vi "Test Validation of CLI arguments.vi"() -> (0 "error out":errorcluster)   [LabVIEW 2025]
doc: "Tests validation of CLI arguments."
uses:
  src/Type Definitions/CLI Argument Setting--cluster.ctl
  <vilib>/addons/_JKI Toolkits/Caraya/classes/Test/Test.lvclass
  <vilib>/addons/_JKI Toolkits/Caraya/classes/Assert/Assert.lvclass
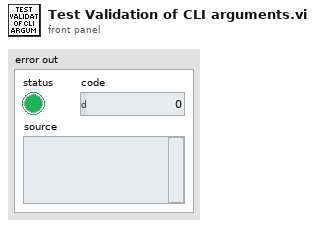
[diagram p1: front panel]
types:
  T1 = typedef "CLI Argument Setting--cluster.ctl" = cluster{"Name Set":bool, "Version Set":bool, "Architecture Set":bool, "File Set":bool}
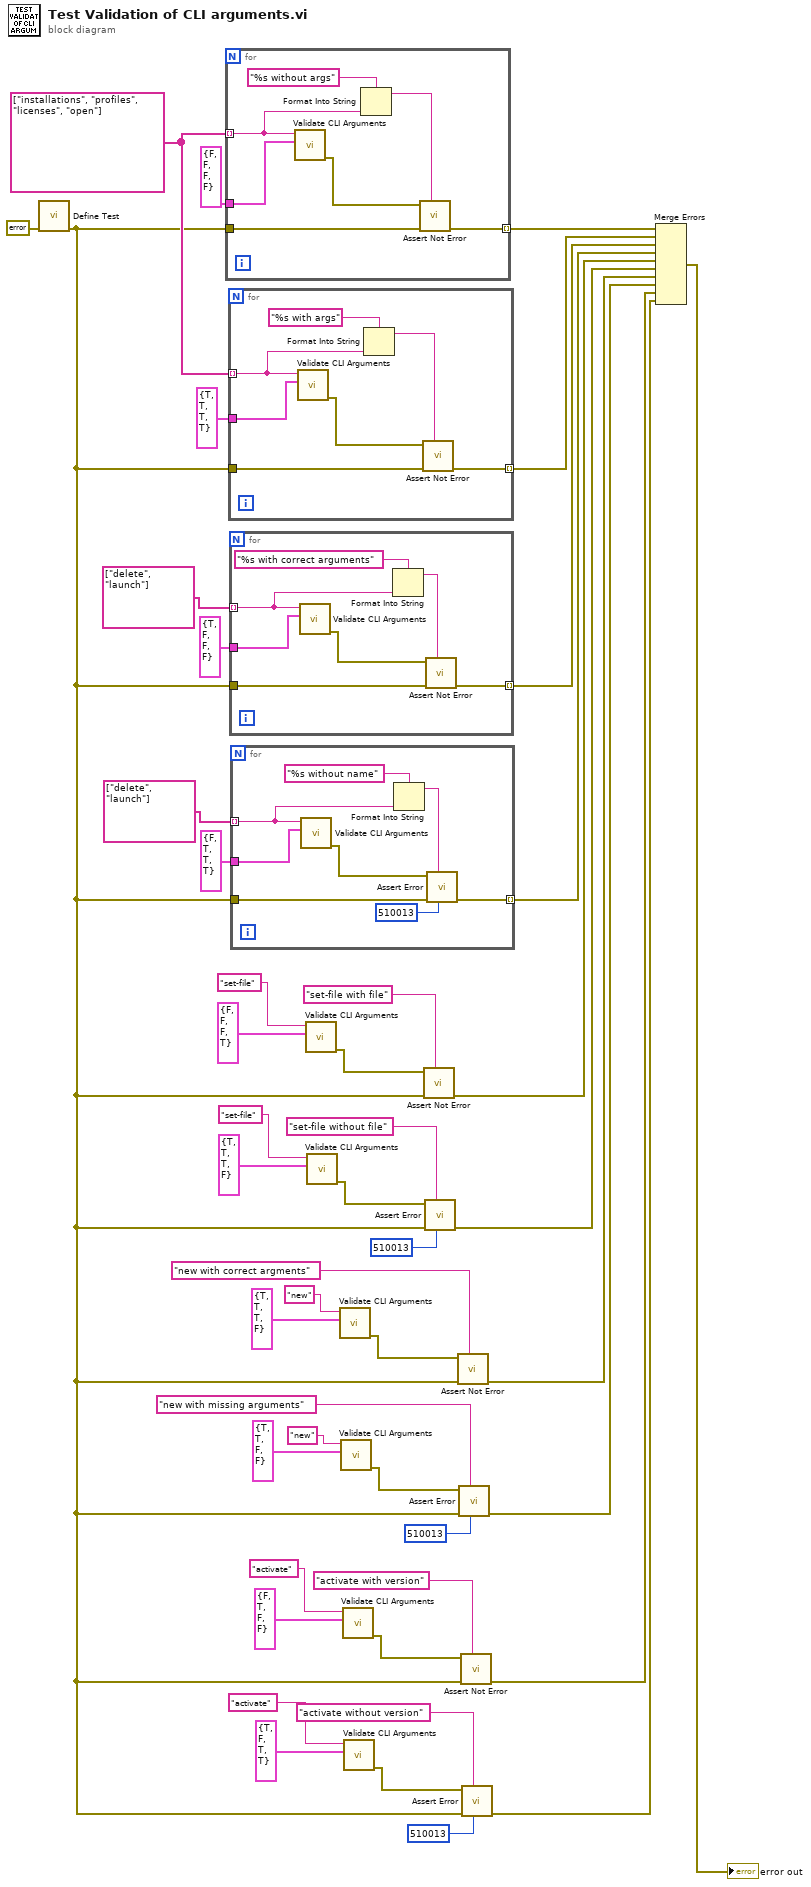
[diagram p0: block diagram]
diagram:
  w46 = string[] ["installations", "profiles", "licenses", "open"]
  n1 = call <vilib>:"Define Test.vi"("error in (no error)"=errorcluster {"status"=FALSE, "code"=0, "source"=""}) -> ("error out"=w3:errorcluster)  [unwired: 9 in, 1 out]
  n2 = for {
    tunnel: w46 -> [w53] mode=indexing
    tunnel: w3 -> [w51]
    tunnel: [w50] -> w26 mode=indexing
    tunnel: T1 {"Name Set"=FALSE, "Version Set"=FALSE, "Architecture Set"=FALSE, "File Set"=FALSE} ("CLI Arguments Setting") -> [w48]
    n3 = call "Validate CLI Arguments.vi"("CLI Arguments Setting"=w48, "Command"=w53) -> ("error out"=w52:errorcluster)  [unwired: 9 in]
    n4 = Format Into String(format string="%s without args" ("Label (VI Title)"), w53) -> (resulting string=w49:string)  [unwired: 2 in, 1 out]
    n5 = call <vilib>:"Assert Not Error.vi"("Label"=w49, "error in (no error)"=w51, "Not Error?"=w52) -> ("error out"=w50:errorcluster)  [unwired: 7 in, 1 out]
  }
  n6 = for {
    tunnel: w46 -> [w60] mode=indexing
    tunnel: w3 -> [w58]
    tunnel: [w57] -> w27 mode=indexing
    tunnel: T1 {"Name Set"=TRUE, "Version Set"=TRUE, "Architecture Set"=TRUE, "File Set"=TRUE} ("CLI Arguments Setting") -> [w55]
    n7 = call "Validate CLI Arguments.vi"("CLI Arguments Setting"=w55, "Command"=w60) -> ("error out"=w59:errorcluster)  [unwired: 9 in]
    n8 = Format Into String(format string="%s with args" ("Label (VI Title)"), w60) -> (resulting string=w56:string)  [unwired: 2 in, 1 out]
    n9 = call <vilib>:"Assert Not Error.vi"("Label"=w56, "error in (no error)"=w58, "Not Error?"=w59) -> ("error out"=w57:errorcluster)  [unwired: 7 in, 1 out]
  }
  n10 = for {
    tunnel: string[] ["delete", "launch"] ("Command") -> [w66] mode=indexing
    tunnel: w3 -> [w64]
    tunnel: [w63] -> w28 mode=indexing
    tunnel: T1 {"Name Set"=TRUE, "Version Set"=FALSE, "Architecture Set"=FALSE, "File Set"=FALSE} ("CLI Arguments Setting") -> [w62]
    n11 = call "Validate CLI Arguments.vi"("CLI Arguments Setting"=w62, "Command"=w66) -> ("error out"=w68:errorcluster)  [unwired: 9 in]
    n12 = Format Into String(format string="%s with correct arguments" ("Label"), w66) -> (resulting string=w65:string)  [unwired: 2 in, 1 out]
    n13 = call <vilib>:"Assert Not Error.vi"("Label"=w65, "error in (no error)"=w64, "Not Error?"=w68) -> ("error out"=w63:errorcluster)  [unwired: 7 in, 1 out]
  }
  n14 = for {
    tunnel: string[] ["delete", "launch"] ("Command") -> [w74] mode=indexing
    tunnel: w3 -> [w72]
    tunnel: [w71] -> w29 mode=indexing
    tunnel: T1 {"Name Set"=FALSE, "Version Set"=TRUE, "Architecture Set"=TRUE, "File Set"=TRUE} ("CLI Arguments Setting") -> [w70]
    n15 = call "Validate CLI Arguments.vi"("CLI Arguments Setting"=w70, "Command"=w74) -> ("error out"=w76:errorcluster)  [unwired: 9 in]
    n16 = Format Into String(format string="%s without name" ("Label"), w74) -> (resulting string=w73:string)  [unwired: 2 in, 1 out]
    n17 = call <vilib>:"Assert Error.vi"("error code (1)"=510013, "Label"=w73, "error in (no error)"=w72, "Error?"=w76) -> ("error out"=w71:errorcluster)  [unwired: 6 in, 1 out]
  }
  n18 = call "Validate CLI Arguments.vi"("CLI Arguments Setting"=T1 {"Name Set"=FALSE, "Version Set"=FALSE, "Architecture Set"=FALSE, "File Set"=TRUE}, "Command"="set-file") -> ("error out"=w40:errorcluster)  [unwired: 9 in]
  n19 = call "Validate CLI Arguments.vi"("CLI Arguments Setting"=T1 {"Name Set"=TRUE, "Version Set"=TRUE, "Architecture Set"=TRUE, "File Set"=FALSE}, "Command"="set-file") -> ("error out"=w36:errorcluster)  [unwired: 9 in]
  n20 = call "Validate CLI Arguments.vi"("CLI Arguments Setting"=T1 {"Name Set"=TRUE, "Version Set"=TRUE, "Architecture Set"=TRUE, "File Set"=FALSE}, "Command"="new") -> ("error out"=w23:errorcluster)  [unwired: 9 in]
  n21 = call "Validate CLI Arguments.vi"("CLI Arguments Setting"=T1 {"Name Set"=TRUE, "Version Set"=TRUE, "Architecture Set"=FALSE, "File Set"=FALSE}, "Command"="new") -> ("error out"=w19:errorcluster)  [unwired: 9 in]
  n22 = call "Validate CLI Arguments.vi"("CLI Arguments Setting"=T1 {"Name Set"=FALSE, "Version Set"=TRUE, "Architecture Set"=FALSE, "File Set"=FALSE}, "Command"="activate") -> ("error out"=w12:errorcluster)  [unwired: 9 in]
  n23 = call "Validate CLI Arguments.vi"("CLI Arguments Setting"=T1 {"Name Set"=TRUE, "Version Set"=FALSE, "Architecture Set"=TRUE, "File Set"=TRUE}, "Command"="activate") -> ("error out"=w8:errorcluster)  [unwired: 9 in]
  n24 = call <vilib>:"Assert Not Error.vi"("Label"="set-file with file", "error in (no error)"=w3, "Not Error?"=w40) -> ("error out"=w30:errorcluster)  [unwired: 7 in, 1 out]
  n25 = call <vilib>:"Assert Error.vi"("error code (1)"=510013, "Label"="set-file without file", "error in (no error)"=w3, "Error?"=w36) -> ("error out"=w31:errorcluster)  [unwired: 6 in, 1 out]
  n26 = call <vilib>:"Assert Not Error.vi"("Label"="new with correct argments", "error in (no error)"=w3, "Not Error?"=w23) -> ("error out"=w13:errorcluster)  [unwired: 7 in, 1 out]
  n27 = call <vilib>:"Assert Error.vi"("error code (1)"=510013, "Label"="new with missing arguments", "error in (no error)"=w3, "Error?"=w19) -> ("error out"=w14:errorcluster)  [unwired: 6 in, 1 out]
  n28 = call <vilib>:"Assert Not Error.vi"("Label"="activate with version", "error in (no error)"=w3, "Not Error?"=w12) -> ("error out"=w1:errorcluster)  [unwired: 7 in, 1 out]
  n29 = call <vilib>:"Assert Error.vi"("error code (1)"=510013, "Label"="activate without version", "error in (no error)"=w3, "Error?"=w8) -> ("error out"=w2:errorcluster)  [unwired: 6 in, 1 out]
  n30 = Merge Errors(w26, w27, w28, w29, w30, w31, w13, w14, w1, w2) -> (→"error out":errorcluster)
